vi "process diagnostic data.vi"(7 "expected slave":i8, 8 "error in":errorcluster, 10 "error specs":T1[](array[typedef]), 11 "diagnostic bytes":u8[](array[numeric]) format="%.0b") -> (0 "error out":errorcluster)   [LabVIEW 2013, in "Profibus Module runtime.lvclass"]
uses:
  Profibus Module runtime.lvclass
  configuration/error throw specification.ctl
  <vilib>/NI/Tag Bus Module Framework/root configuration/TBM configuration.lvclass
  configuration/Profibus Module configuration.lvclass
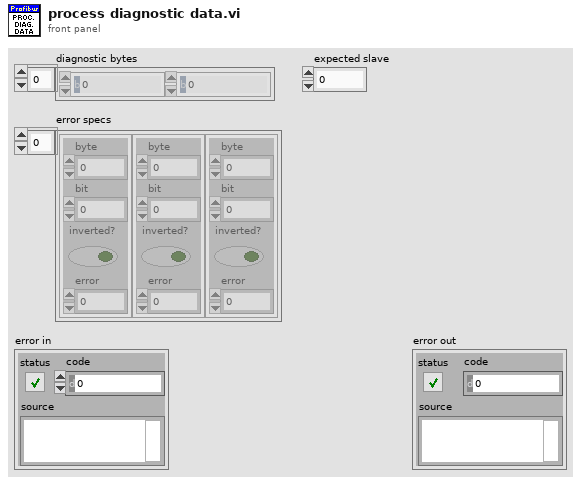
[diagram p1: front panel]
types:
  T1 = typedef "Profibus Module configuration.lvclass/error throw specification.ctl" = cluster{"byte":i32, "bit":i32, "inverted?":bool, "error":i32}
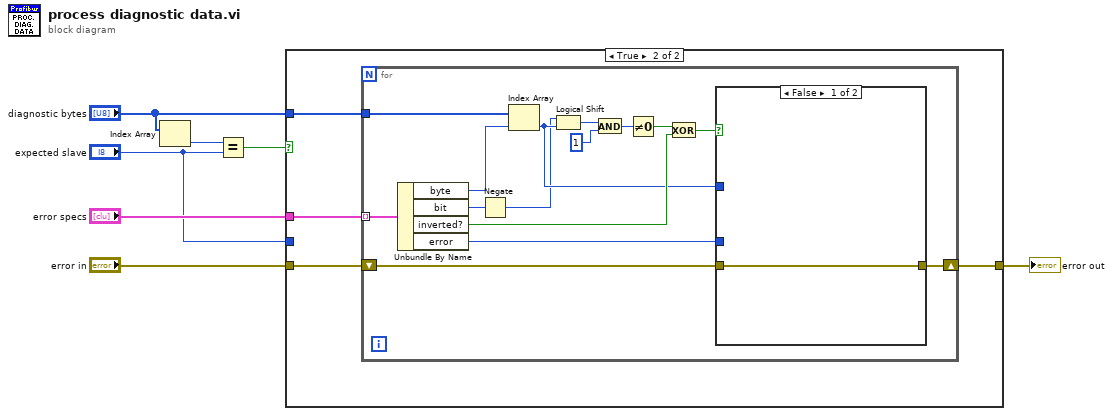
[diagram p0: block diagram]
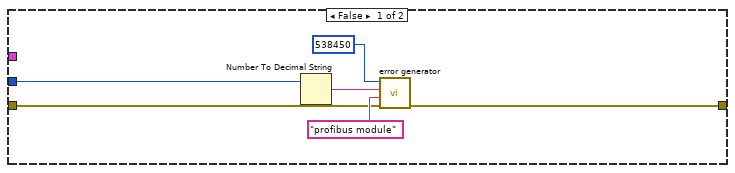
[diagram p2: hidden frame]
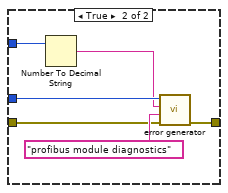
[diagram p3: hidden frame]
diagram:
  n1 = Index Array(array="diagnostic bytes") -> (element=w5:u8)  [unwired: 1 in]
  n2 = Equal?(x=w5, y="expected slave") -> (x = y?=w4:bool)
  n3 = case shown="True" w4 {
    tunnel: "error specs" -> [_ w17]
    tunnel: "diagnostic bytes" -> [_ w16]
    tunnel: [w10 w14] -> w3
    tunnel: "error in" -> [w9 w15]
    tunnel: "expected slave" -> [w8 _]
    frame False {
      n4 = Number To Decimal String(number=w8) -> (decimal integer string=w12:string)  [unwired: 1 in]
      n5 = call <vilib>:"error generator.vi"("error in"=w9, "source"="profibus module", "append error message"=w12, "error code (0)"=538450) -> ("error out"=w10:errorcluster)  [unwired: 7 in]
    }
    frame True {
      n6 = for {
        tunnel: w17 -> [w32] mode=indexing
        tunnel: w16 -> [w31]
        shift-right: [w20] -> w14
        shift-left: w15 -> [w21]
        n7 = Unbundle By Name(w32) -> ("byte"=w30:i32, "bit"=w29:i32, "inverted?"=w24:bool, "error"=w22:i32)
        n8 = Negate(x=w29) -> (-x=w18:i32)
        n9 = Index Array(array=w31, index=w30) -> (element=w19:u8)
        n10 = Logical Shift(y=w18, x=w19) -> (x << y=w28:u8)
        n11 = And(x=w28, y=u8 1) -> (x .and. y?=w26:u8)
        n12 = Not Equal To 0?(x=w26) -> (x != 0?=w25:bool)
        n13 = Exclusive Or(1:w24, 2:w25) -> (0:w23:bool)
        n14 = case shown="False" w23 {
          tunnel: w22 -> [_ w36]
          tunnel: w21 -> [w33 w38]
          tunnel: [w33 w37] -> w20
          tunnel: w19 -> [_ w35]
          frame False {
          }
          frame True {
            n15 = Number To Decimal String(number=w35) -> (decimal integer string=w34:string)  [unwired: 1 in]
            n16 = call <vilib>:"error generator.vi"("error in"=w38, "source"="profibus module diagnostics", "append error message"=w34, "error code (0)"=w36) -> ("error out"=w37:errorcluster)  [unwired: 7 in]
          }
        }
      }
    }
  }
  "error out" <- w3
